vi "Waveform Attribute, Get MD5.vi"(6 "error in":errorcluster, 9 "waveform":waveform(dbl)) -> (0 "error out":errorcluster, 3 "waveform dup":waveform(dbl), 4 "MD5":string)   [LabVIEW 2010]
doc: "This function retrieves an MD5 message-digest from waveform attributes.\n\nThe message digest string is assembled from four attributes stored as double precision floating point values (MD5[0], MD5[1], MD5[2, and MD5[3]).\n\nThe inverse of this function is \"MD5, Waveform Attribute, Set MD5.vi\""
panel:
  out "MD5[3]":dbl=nan format="%.1f"
  out "MD5[2]":dbl=nan format="%.1f"
  out "MD5[1]":dbl=nan format="%.1f"
  out "MD5[0]":dbl=nan format="%.1f"
  # "Waveform Attributes"
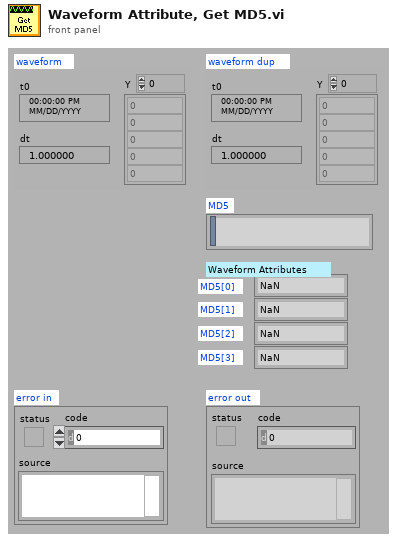
[diagram p1: front panel]
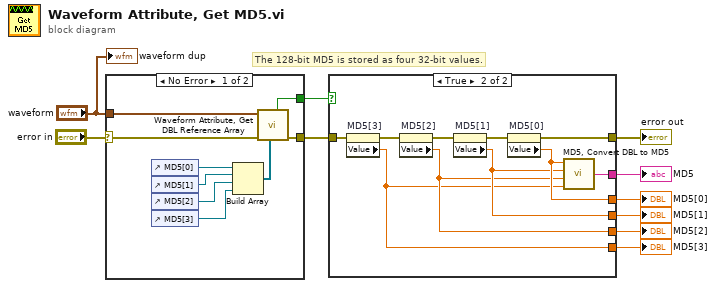
[diagram p0: block diagram]
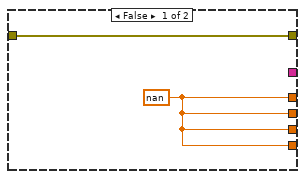
[diagram p3: hidden frame]
diagram:
  # "The 128-bit MD5 is stored as four 32-bit values."
  n1 = case shown="No Error" "error in" {
    selector: "error in" -> [w13 w20]
    tunnel: [w14 w20] -> w1
    tunnel: "waveform" -> [w12 _]
    tunnel: [w11 _] -> w2
    frame No Error {
      n2 = control-ref of="MD5[0]"() -> (w15:refnum<vi>)
      n3 = control-ref of="MD5[1]"() -> (w16:refnum<vi>)
      n4 = control-ref of="MD5[2]"() -> (w17:refnum<vi>)
      n5 = control-ref of="MD5[3]"() -> (w18:refnum<vi>)
      n6 = Build Array(w15, w16, w17, w18) -> (w19:refnum<vi>[])
      n7 = call "Waveform Attribute, Get DBL Reference Array.vi"("refnum array"=w19, "error in"=w13, "waveform"=w12) -> ("error out"=w14:errorcluster, "found all values"=w11:bool)  [unwired: 2 in, 3 out]
    }
    frame Error {
    }
  }
  n8 = case shown="True" w2 {
    tunnel: [w21 w29] -> w10
    tunnel: [_ w28] -> w9
    tunnel: [w22 w27] -> w8
    tunnel: [w22 w26] -> w7
    tunnel: [w22 w25] -> w6
    tunnel: [w22 w24] -> w5
    tunnel: w1 -> [w21 w23]
    frame False {
      w22 = nan ("Value")
    }
    frame True {
      n9 = property on="MD5[3]" class="DigNum (strict)"(error in=w23) -> (error out=w32:errorcluster, "Value"=w24:dbl)  [unwired: 1 in, 1 out]
      n10 = property on="MD5[2]" class="DigNum (strict)"(error in=w32) -> (error out=w31:errorcluster, "Value"=w25:dbl)  [unwired: 1 in, 1 out]
      n11 = property on="MD5[1]" class="DigNum (strict)"(error in=w31) -> (error out=w30:errorcluster, "Value"=w26:dbl)  [unwired: 1 in, 1 out]
      n12 = property on="MD5[0]" class="DigNum (strict)"(error in=w30) -> (error out=w29:errorcluster, "Value"=w27:dbl)  [unwired: 1 in, 1 out]
      n13 = call "MD5, Convert DBL to MD5.vi"("MD5[0]"=w27, "MD5[1]"=w26, "MD5[2]"=w25, "MD5[3]"=w24) -> ("MD5"=w28:string)  [unwired: 1 out]
    }
  }
  "error out" <- w10
  "MD5" <- w9
  "MD5[0]" <- w8
  "MD5[1]" <- w7
  "MD5[2]" <- w6
  "MD5[3]" <- w5
  "waveform dup" <- "waveform"
